vi "OpenTcpMessageConnection.vi"(6 "timeout (ms)":i32=-1, 8 "error in (no error)":errorcluster, 9 "Port":u16, 10 "Hostname":string, 11 "ClientName":string) -> (0 "error out":errorcluster, 3 "connection ID out":T1)   [LabVIEW 2017]
uses:
  <vilib>/addons/InsightCM/MessageBus/TcpApi/controls/TcpMessageReference.ctl
  <vilib>/addons/InsightCM/MessageBus/TcpApi/controls/TcpMessageReferenceData.ctl
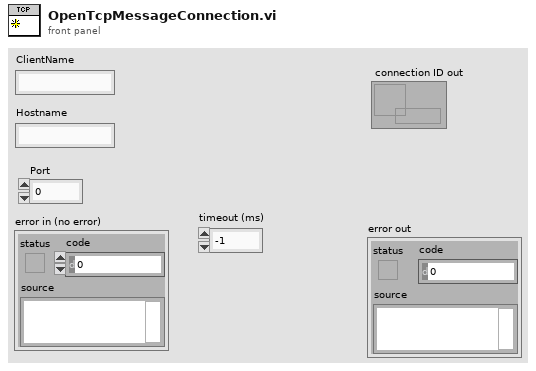
[diagram p1: front panel]
types:
  T1 = typedef "TcpMessageReference.ctl" = refnum<data-value>
  T2 = typedef "TcpMessageReferenceData.ctl" = cluster{"ClientName":string, "CmdStream":refnum<k5>, "FileStream":refnum<k5>}
  T3 = cluster{"AuthDeviceGUID":string, "ClientName":string}
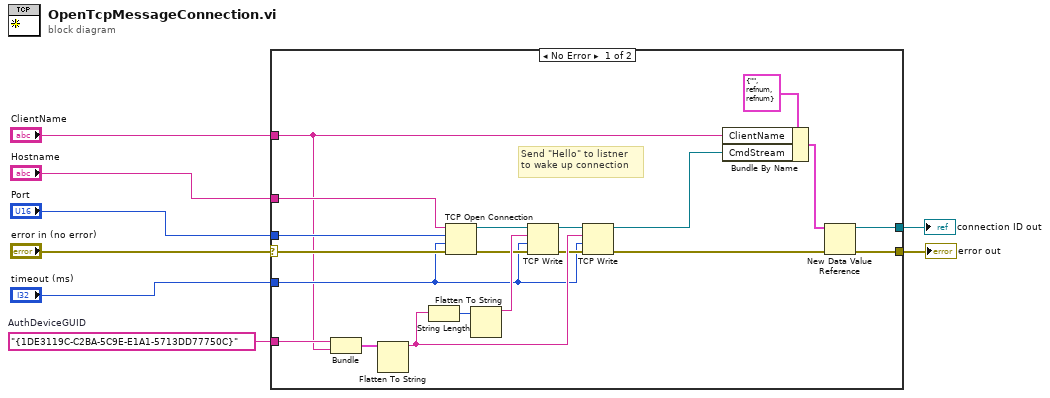
[diagram p0: block diagram]
diagram:
  w4 = "{1DE3119C-C2BA-5C9E-E1A1-5713DD77750C}"  # AuthDeviceGUID
  n1 = case shown="No Error" "error in (no error)" {
    selector: "error in (no error)" -> [w16 w29]
    tunnel: [w17 w29] -> w1
    tunnel: "timeout (ms)" -> [w13 _]
    tunnel: "Port" -> [w12 _]
    tunnel: "Hostname" -> [w19 _]
    tunnel: "ClientName" -> [w11 _]
    tunnel: w4 -> [w14 _]
    tunnel: [w15 _] -> w2
    frame No Error {
      # "Send \"Hello\" to listner\nto wake up connection"
      n2 = Bundle("AuthDeviceGUID"=w14, "ClientName"=w11) -> (w20:T3)  [unwired: 1 in]
      n3 = Flatten To String(anything=w20) -> (data string=w27:string)  [unwired: 3 in, 2 out]
      n4 = String Length(string=w27) -> (length=w25:i32)
      n5 = TCP Open Connection(address=w19, remote port or service name=w12, timeout ms (60000)=w13, error in (no error)=w16) -> (connection ID=w22:refnum<k5>, error out=w23:errorcluster)  [unwired: 1 in]
      n6 = Flatten To String(anything=w25) -> (data string=w26:string)  [unwired: 3 in, 2 out]
      n7 = TCP Write(connection ID=w22, data in=w26, error in (no error)=w23, 9:w13) -> (connection ID out=w28:refnum<k5>, error out=w24:errorcluster)  [unwired: 1 out]
      n8 = TCP Write(connection ID=w28, data in=w27, error in (no error)=w24, 9:w13) -> (connection ID out=w10:refnum<k5>, error out=w9:errorcluster)  [unwired: 1 out]
      n9 = Bundle By Name(cluster=T2 {"ClientName"="", "CmdStream"=refnum, "FileStream"=refnum} ("data value"), "ClientName"=w11, "CmdStream"=w10) -> (w18:T2)
      n10 = New Data Value Reference(data value=w18, error in=w9) -> (data value reference=w15:refnum<data-value>, error out=w17:errorcluster)
    }
    frame Error {
    }
  }
  "connection ID out" <- w2
  "error out" <- w1
